vi "Input supports bracketed too.vi"(8 "error in (no error)":errorcluster, 10 "Text.Font:Size":u32, 11 "User Message":string) -> (0 "error out":errorcluster, 3 "Data out":string)   [LabVIEW 2013]
doc: "Run the VI to and press keys on the keyboard. \nThe Key Released VI reports the value of the key up event."
panel:
  in  "Data":string
  out "Key pressed from array":string
  out "Key released":string
  in  "stop":bool
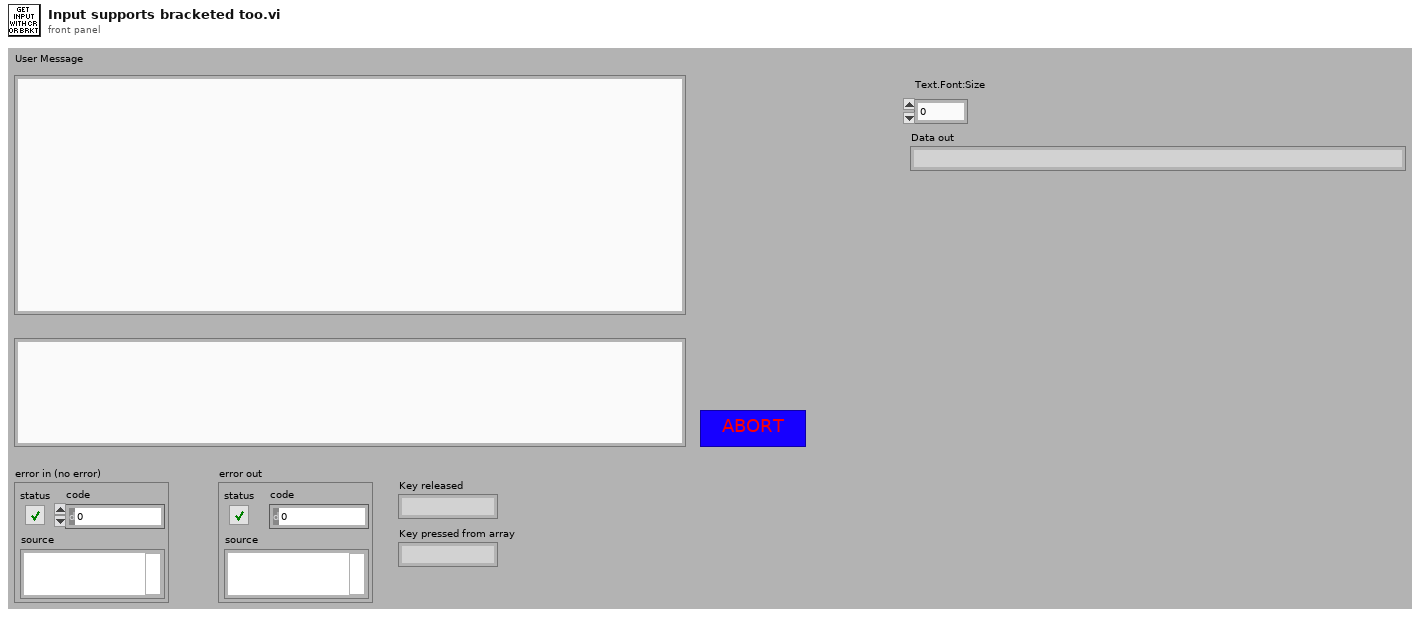
[diagram p1: front panel]
types:
  T1 = cluster{"Shift":bool, "Ctrl":bool, "Alt":bool, "Cmd":bool, "Opt":bool}
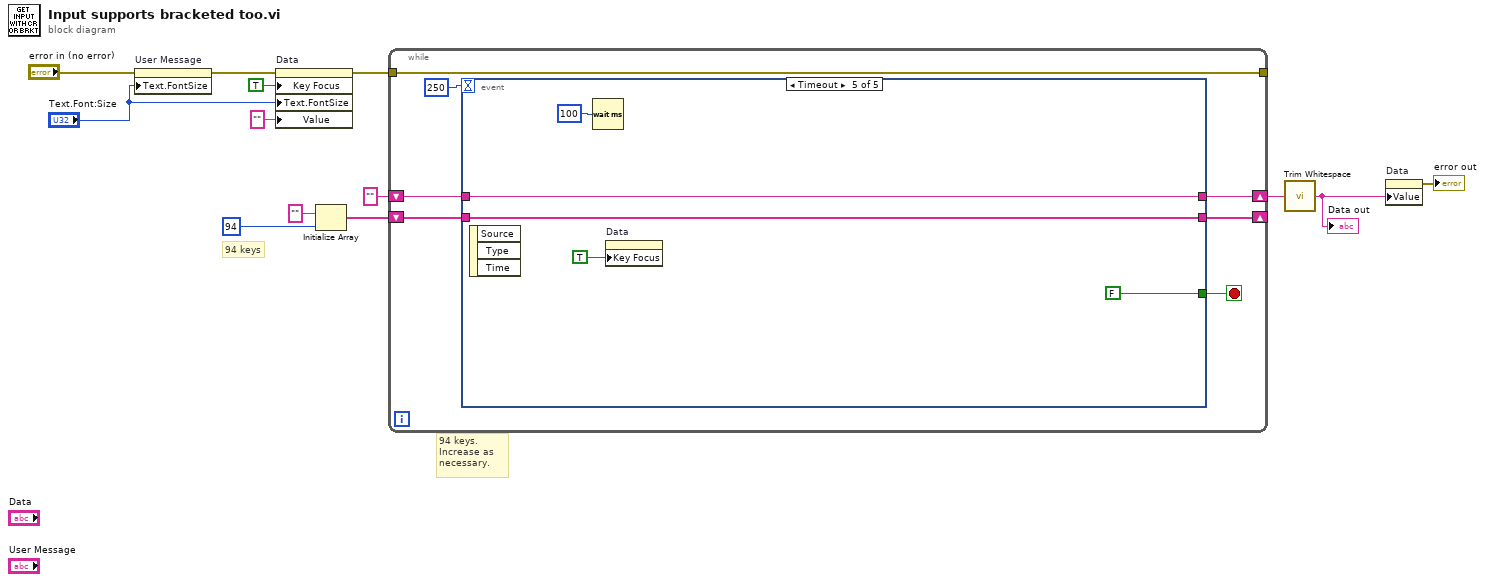
[diagram p0: block diagram]
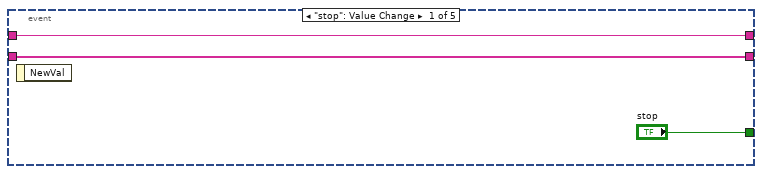
[diagram p2: hidden frame]
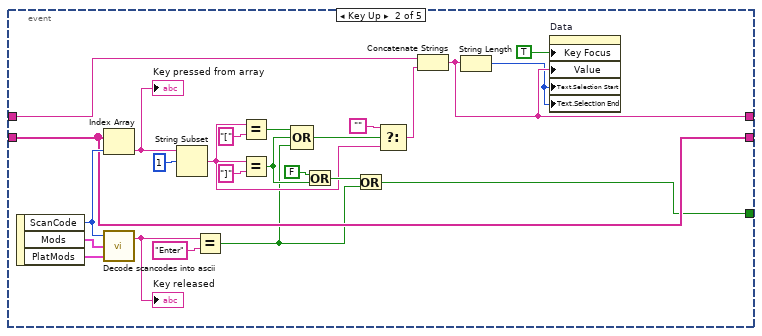
[diagram p3: hidden frame]
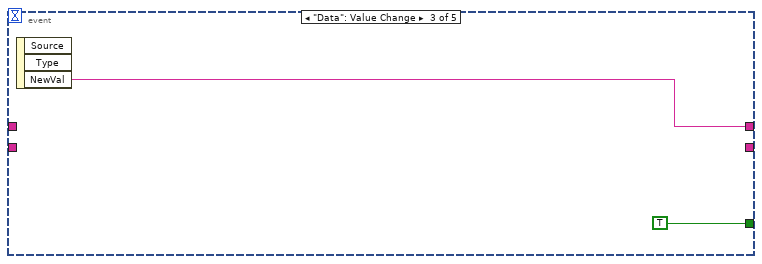
[diagram p4: hidden frame]
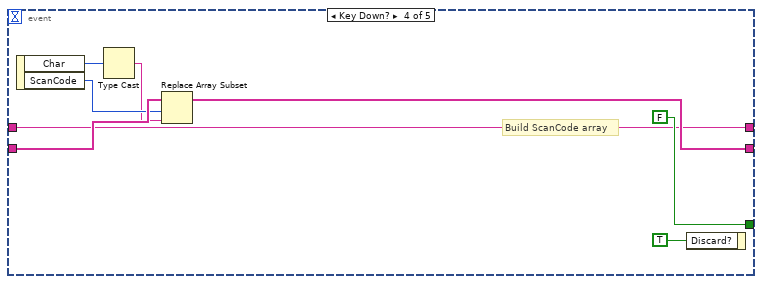
[diagram p5: hidden frame]
diagram:
  # "94 keys. Increase as necessary."
  # "94 keys"
  n1 = property on="User Message" class="Str"(error in="error in (no error)", "Text.FontSize"="Text.Font:Size") -> (error out=w9:errorcluster)  [unwired: 1 in, 1 out]
  n2 = property on="Data" class="Str"(error in=w9, "Key Focus"=TRUE, "Text.FontSize"="Text.Font:Size", "Value"="" ("Data")) -> (error out=w8:errorcluster)  [unwired: 1 in, 1 out]
  n3 = Initialize Array("", 94) -> (w13:string[])
  n4 = while {
    shift-right: [w18] -> _
    shift-left: w13 -> [w19]
    shift-right: [w16] -> w4
    shift-left: "" -> [w17]
    tunnel: [w15] -> _
    tunnel: w8 -> [w15]
    stop <- w20 stop-if-true
    n5 = event shown="[4] Timeout" {
      selector: _ -> [_ _ _ _ _]
      dyn-events: _ -> [_ _ _ _ _]
      timeout: 250 -> [_ _ _ _ _]
      tunnel: ["stop" w35 TRUE ("stop") FALSE FALSE ("stop")] -> w20
      tunnel: w19 -> [w22 w44 _ w57 w61]
      tunnel: [w22 w44 _ w54 w61] -> w18
      tunnel: w17 -> [w21 w43 _ w50 w60]
      tunnel: [w21 w26 w49 w50 w60] -> w16
      event "stop": Value Change {
        n6 = event-data() -> ()  [unwired: 1 in, 1 out]
      }
      event Key Up {
        n7 = event-data() -> ("ScanCode"=w45:i16, "Mods"=w46:cluster{"Num Pad":bool, "Menu Key":bool}, "PlatMods"=w47:T1)  [unwired: 1 in]
        n8 = Index Array(array=w44, index=w45) -> (element=w40:string)
        "Key pressed from array" <- w40
        n9 = call "Decode scancodes into ascii.vi"("PlatMods"=w47, "Mods"=w46, "ScanCode"=w45) -> ("String"=w38:string)  [unwired: 1 out]
        "Key released" <- w38
        n10 = String Subset(string=w40, offset (0)=1) -> (substring=w31:string)  [unwired: 1 in]
        n11 = Equal?(x=w38, y="Enter") -> (x = y?=w28:bool)
        n12 = Equal?(x=w31, y="[") -> (x = y?=w30:bool)
        n13 = Equal?(x=w31, y="]") -> (x = y?=w29:bool)
        n14 = Compound Arithmetic op=OR(w30, w29, w28) -> (w27:bool)
        n15 = Or(x=FALSE, y=w29) -> (x .or. y?=w36:bool)
        n16 = Or(x=w36, y=w28) -> (x .or. y?=w35:bool)
        n17 = Select(t="", s=w27, f=w31) -> (s? t:f=w33:string)
        n18 = Concatenate Strings(w43, w33) -> (w26:string)
        n19 = String Length(string=w26) -> (length=w25:i32)
        n20 = property on="Data" class="Str"("Key Focus"=TRUE, "Value"=w26, "Text.Selection Start"=w25, "Text.Selection End"=w25) -> ()  [unwired: 2 in, 2 out]
      }
      event "Data": Value Change {
        n21 = event-data() -> ("NewVal"=w49:string)  [unwired: 1 in, 2 out]
      }
      event Key Down? {
        # "Build ScanCode array"
        n22 = event-data() -> ("Char"=w55:i16, "ScanCode"=w56:i16)  [unwired: 1 in]
        n23 = Type Cast(x=w55) -> (*(type *) &x=w53:string)  [unwired: 1 in]
        n24 = Replace Array Subset(array=w57, new element=w53, index=w56) -> (w54:string[])
        n25 = event-data("Discard?"=TRUE) -> ()  [unwired: 1 in, 1 out]
      }
      event Timeout {
        n26 = event-data() -> ()  [unwired: 1 in, 3 out]
        n27 = Wait (ms)(milliseconds to wait=u32 100) -> ()  [unwired: 1 out]
        n28 = property on="Data" class="Str"("Key Focus"=TRUE) -> ()  [unwired: 2 in, 2 out]
      }
    }
  }
  n29 = call <vilib>:"Trim Whitespace.vi"("string"=w4) -> ("trimmed string"=w2:string)  [unwired: 1 in]
  "Data out" <- w2
  n30 = property on="Data" class="Str"("Value"=w2) -> (error out=→"error out":errorcluster)  [unwired: 2 in, 1 out]
